vi "Read Item Path.vi"(8 "error in (no error)":errorcluster, 11 "MenuSelectionMsg in":refnum<class "MenuSelectionMsg.lvclass">) -> (0 "error out":errorcluster, 2 "Item Path":string, 3 "MenuSelectionMsg out":refnum<class "MenuSelectionMsg.lvclass">)   [LabVIEW 2017, in "ActorEvents.lvlib" / "MenuSelectionMsg.lvclass"]
uses:
  MenuSelectionMsg.lvclass
  MenuSelectionMsg.lvclass/MenuSelectionMsg.ctl
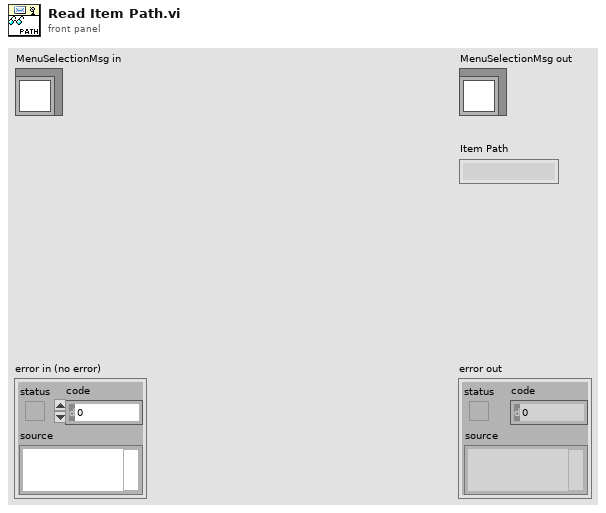
[diagram p1: front panel]
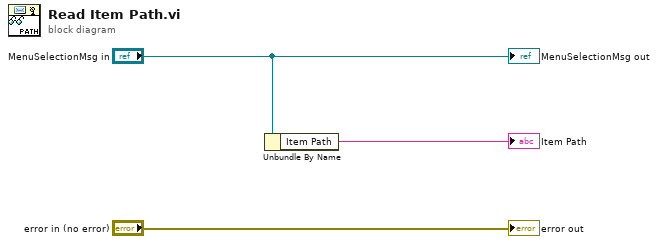
[diagram p0: block diagram]
diagram:
  n1 = Unbundle By Name("MenuSelectionMsg in") -> ("Item Path"=→"Item Path":string)
  "error out" <- "error in (no error)"
  "MenuSelectionMsg out" <- "MenuSelectionMsg in"
